vi "AD7609_Init.vi"() -> (0 "OK":bool)   [LabVIEW 2012]
uses:
  glADC.vi
  <vilib>/rvi/eio/common/nirviEmuTemplateMethod_errors.vi
  <vilib>/eio/EIONode/EIONode.xnode
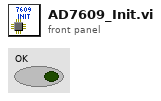
[diagram p1: front panel]
types:
  T1 = cluster{"OS":u8, "Range":u8, "T_hi":u8, "D_low":u8}
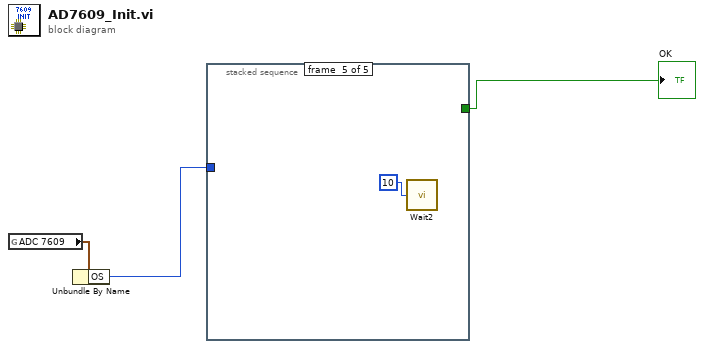
[diagram p0: block diagram]
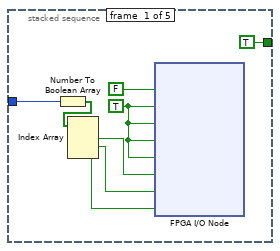
[diagram p2: hidden frame]
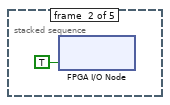
[diagram p3: hidden frame]
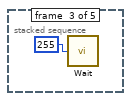
[diagram p4: hidden frame]
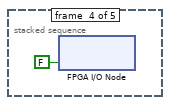
[diagram p5: hidden frame]
diagram:
  n1 = global read "glADC.vi" "ADC 7609"() -> (w2:T1)
  n2 = Unbundle By Name(w2) -> ("OS"=w1:u8)
  n3 = stacked-sequence {
    tunnel: [TRUE ("RESET") _ _ _ _] -> w3
    tunnel: w1 -> [w6 _ _ _ _]
    frame #0 {
      w4 = TRUE ("CONVST")
      n4 = Number To Boolean Array(number=w6) -> (Boolean array=w10:bool[])
      n5 = Index Array(array=w10) -> (element #1=w9:bool, element #2=w8:bool, element #3=w7:bool)  [unwired: 3 in]
      n6 = xnode "FPGA I/O Node"("RESET"=FALSE, "CONVST1"=w4, "CONVST2"=w4, "RD1"=w4, "RD2"=w4, "OS0"=w9, "OS1"=w8, "OS2"=w7) -> ()  [unwired: 8 in, 8 out]
    }
    frame #1 {
      n7 = xnode "FPGA I/O Node"("RESET"=TRUE) -> ()  [unwired: 1 in, 1 out]
    }
    frame #2 {
      n8 = call "Wait"("Count(Ticks)"=u8 255 ("T_reset")) -> ()  [unwired: 1 out]
    }
    frame #3 {
      n9 = xnode "FPGA I/O Node"("RESET"=FALSE) -> ()  [unwired: 1 in, 1 out]
    }
    frame #4 {
      n10 = call "Wait2"("Count(Ticks)"=u8 10 ("D_reset")) -> ()  [unwired: 1 out]
    }
  }
  "OK" <- w3
